vi "Teleop.vi"(10 "Match Info":T3={"Autonomous Elapsed Seconds"=0.0, "TeleOp Elapsed Seconds"=0.0, "Disabled Elapsed Seconds"=0.0, "Visited Autonomous"=FALSE, "Visited TeleOp"=FALSE, "Visited Disabled"=FALSE, "Autonomous Settings"={"Autonomous Style"=enum."Independent", "VI Refnum"=refnum}}, 11 "Call Context":T4) -> ()   [LabVIEW 2013]
doc: "This VI is called for each TeleOp packet received from the DS where the robot is not disabled. It is often used to read from the joysticks and update I/O or to update setpoints for timed control loops. It should complete and return within 20 milliseconds or it may miss DS packets."
uses:
  <vilib>/Rock Robotics/WPI/DriverStation/WPI_DriverStationDerivedRobotMode.ctl
  <vilib>/Rock Robotics/WPI/DriverStation/WPI_DriverStationMatch Info.ctl
  <vilib>/Rock Robotics/WPI/Solenoid/WPI_SolenoidValue.ctl
  Robot Global Data.vi
  <vilib>/Rock Robotics/WPI/Joystick/WPI_JoystickGetSetRefNum.vi
  <vilib>/Rock Robotics/WPI/Solenoid/WPI_SolenoidSetEnum.vi
  <vilib>/Rock Robotics/WPI/RobotDrive/WPI_RobotDriveGetSetRefNum.vi
  <vilib>/addons/control/pid/NI_PID_pid.lvlib
  <vilib>/addons/control/pid/pid.llb/PID (DBL).vi
panel:
  in  "Shooter Motor":dbl(slide) scale=-1.0..1.0
  in  "PID gains Anglerometer":T1={"proportional gain (Kc)"=1.0, "integral time (Ti, min)"=0.01, "derivative time (Td, min)"=0.0} {"derivative time (Td, min)" format="%.3f"; "integral time (Ti, min)" format="%.3f"; "proportional gain (Kc)" format="%.3f"}
  out "Shooter Angle":dbl
  out "Shooter At Target Angle":bool
  out "Cim Speed":dbl
  out "Time For Shooter":dbl
  in  "shooter state":T2(ring)
  out "Numeric 1":dbl(slide) scale=0.0..100.0
  out "Boolean 2":bool
  out "Boolean 1":bool
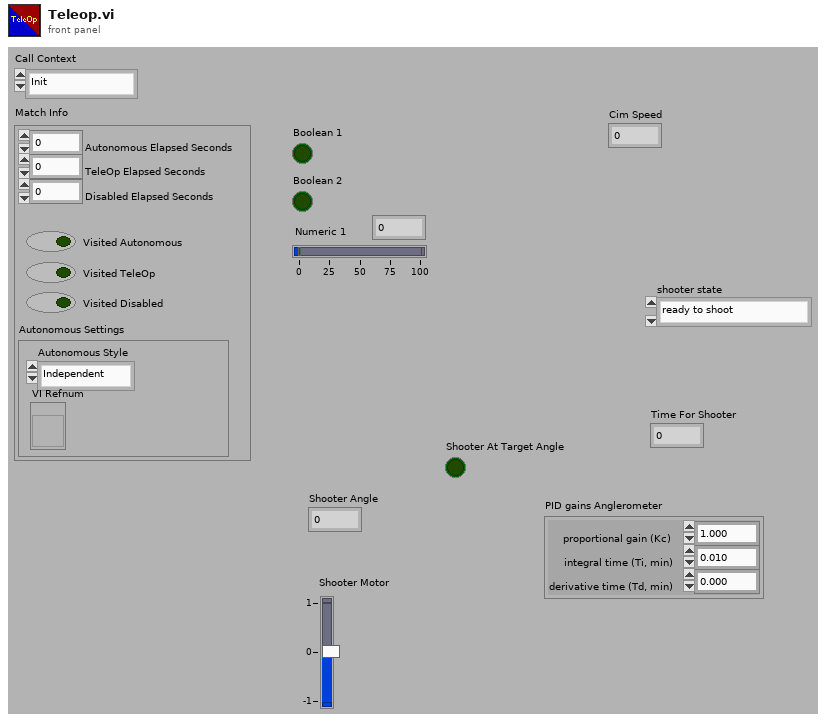
[diagram p1: front panel]
types:
  T1 = cluster{"proportional gain (Kc)":dbl, "integral time (Ti, min)":dbl, "derivative time (Td, min)":dbl}
  T2 = enum16{"ready to shoot", "shooting", "reloading"}
  T3 = typedef "WPI_DriverStationMatch Info.ctl" = cluster{"Autonomous Elapsed Seconds":dbl, "TeleOp Elapsed Seconds":dbl, "Disabled Elapsed Seconds":dbl, "Visited Autonomous":bool, "Visited TeleOp":bool, "Visited Disabled":bool, "Autonomous Settings":cluster{"Autonomous Style":enum16{"Iterative", "Independent"}, "VI Refnum":refnum<vi>}}
  T4 = typedef "WPI_DriverStationDerivedRobotMode.ctl" = enum16{"Init", "Execute", "Stop"}
  T5 = typedef "WPI_PWMDeviceRef.ctl" = cluster{"DeviceStatus":errorcluster, "Digital Module":T6, "PWM Channel":T7}
  T6 = typedef "FPGA_TypedefDigitalModule.ctl" = enum16{"Digital Module 1", "Digital Module 2"}
  T7 = typedef "FPGA_DIOPWMChannel.ctl" = enum8{"PWM 1", "PWM 2", "PWM 3", "PWM 4", "PWM 5", "PWM 6", "PWM 7", "PWM 8", "PWM 9", "PWM 10", "Invalid"}
  T8 = typedef "WPI_MotorControlDeviceRef.ctl" = cluster{"DeviceStatus":errorcluster, "Type":enum16{"PWM", "CAN"}, "PWM":cluster{"Digital Module":T6, "PWM Channel":T7, "DeadBand":T9}, "CAN":cluster{"Device Number":u8, "Control Mode":T10, "Semaphore":T11, "Max Vout":dbl}, "Invert":bool, "TransformRef":T12, "InvTransformRef":T12}
  T9 = typedef "WPI_PWMDeadband.ctl" = cluster{"Name":string, "maxPositivePwm":i32, "minPositivePwm":i32, "centerPwm":i32, "maxNegativePwm":i32, "minNegativePwm":i32, "angularRange":u16}
  T10 = typedef "WPI_CANJaguar_ControlMode.ctl" = enum8{"Percent VBus", "Current", "Speed", "Position", "Voltage"}
  T11 = typedef "Semaphore RefNum" = refnum<k1>
  T12 = typedef "WPI_PWMTransform_ConPane.ctl" = refnum<vi>
  T13 = typedef "WPI_RobotDriveDevRef.ctl" = cluster{"DevStatus":errorcluster, "Motors[]":T8[], "Square Inputs":bool, "Max Output":dbl, "Isochronous":bool}
  T14 = typedef "WPI_JoystickDevRef.ctl" = cluster{"Device":T15}
  T15 = typedef "WPI_JoystickDeviceEnum.ctl" = enum16{"USB 1", "USB 2", "USB 3", "USB 4", "Kinect 1", "Kinect 2"}
  T16 = typedef "WPI_JoystickButtonState.ctl" = cluster{"Button 1":bool, "Button 2":bool, "Button 3":bool, "Button 4":bool, "Button 5":bool, "Button 6":bool, "Button 7":bool, "Button 8":bool, "Button 9":bool, "Button 10":bool, "Button 11":bool, "Button 12":bool}
  T17 = cluster{"axis 1 (x)":dbl, "axis 2 (y)":dbl, "axis 3 (throttle)":dbl, "axis 4":dbl, "axis 5":dbl, "axis 6":dbl}
  T18 = typedef "WPI_SolenoidValue.ctl" = enum16{"Off", "On", "Forward", "Reverse"}
  T19 = typedef "WPI_SolenoidDevRef.ctl" = cluster{"DevStatus":errorcluster, "Solenoid Module":T20, "Forward Solenoid Channel":T21, "Reverse Solenoid Channel":T21}
  T20 = typedef "FPGA_TypedefSolenoidModule.ctl" = enum16{"Solenoid Module 1", "Solenoid Module 2"}
  T21 = typedef "WPI_SolenoidChannel.ctl" = enum8{"Solenoid 1", "Solenoid 2", "Solenoid 3", "Solenoid 4", "Solenoid 5", "Solenoid 6", "Solenoid 7", "Solenoid 8", "Invalid"}
  T22 = typedef "WPI_EncoderDevRef.ctl" = cluster{"DevStatus":errorcluster, "EncoderIndex":T23, "CounterIndex":T24, "DistancePerCount":dbl, "Decoding Type":T25}
  T23 = typedef "FPGA_EncoderIdx.ctl" = enum8{"Enc 0", "Enc 1", "Enc 2", "Enc 3", "Invalid"}
  T24 = typedef "FPGA_CounterCtrSystemIndex.ctl" = enum8{"Ctr 0", "Ctr 1", "Ctr 2", "Ctr 3", "Ctr 4", "Ctr 5", "Ctr 6", "Ctr 7", "Invalid"}
  T25 = typedef "WPI_EncoderType.ctl" = enum16{"1x", "2x", "4x"}
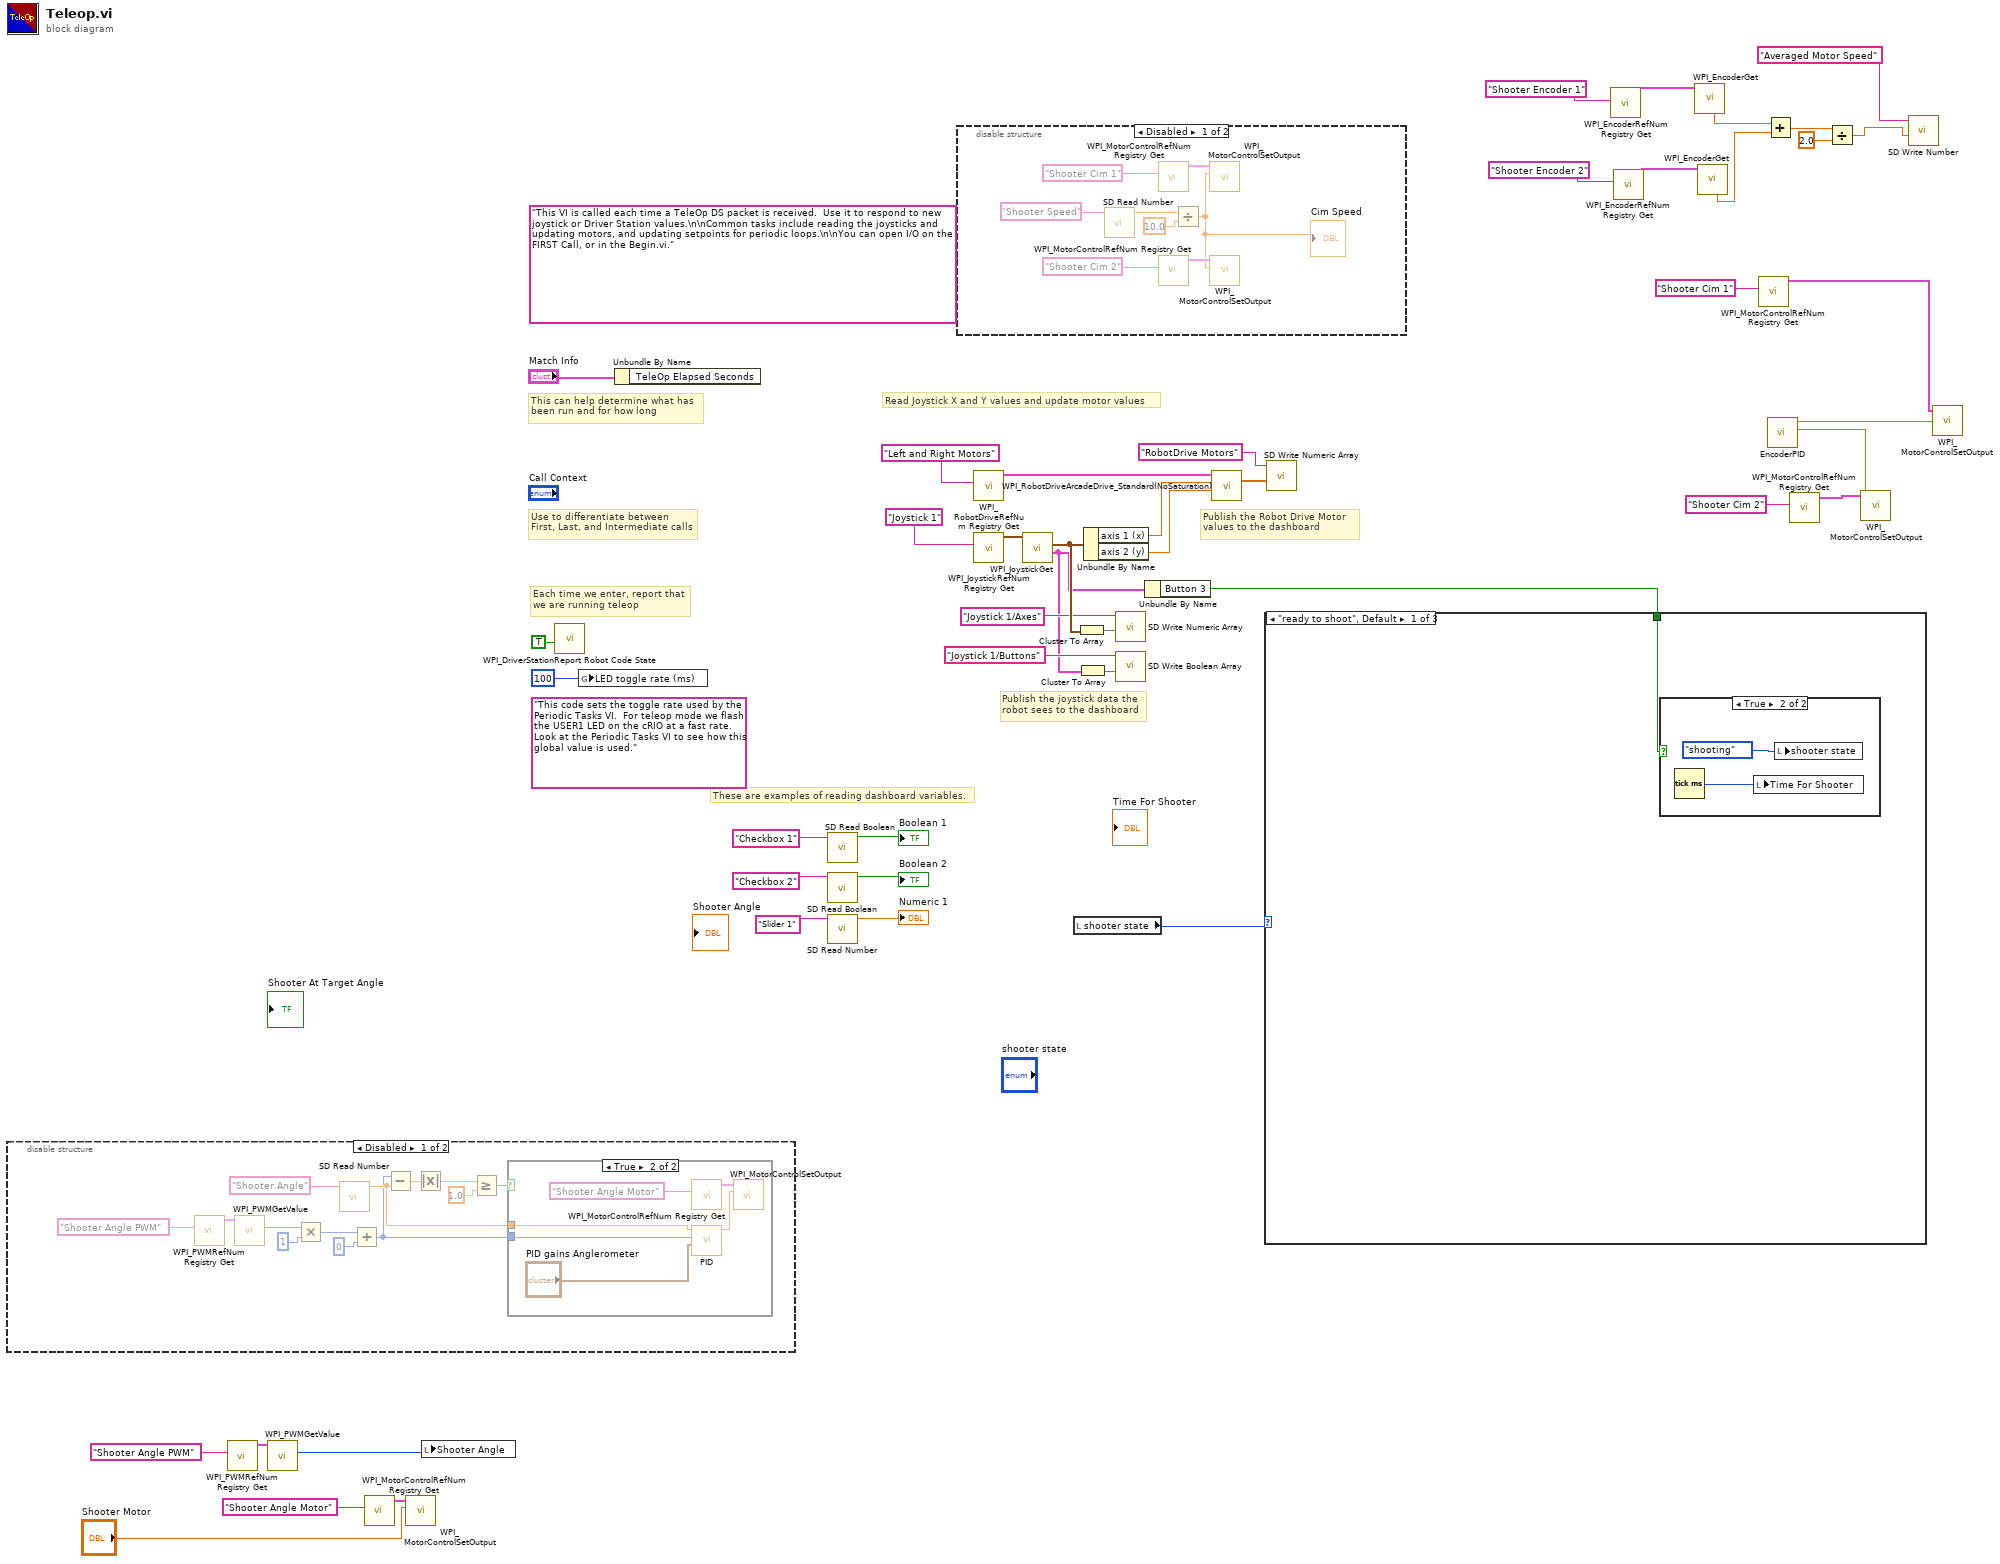
[diagram p0: block diagram]
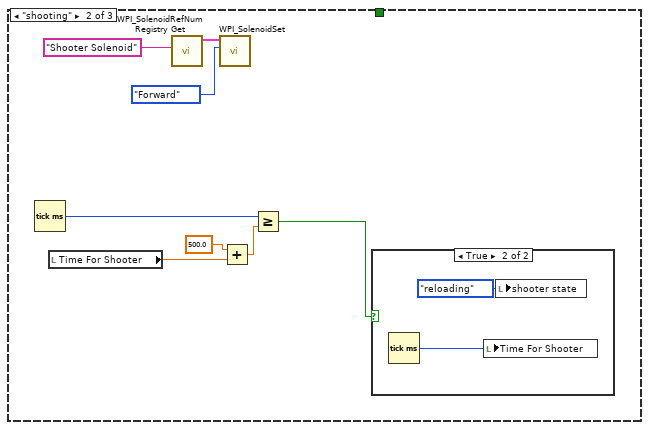
[diagram p6: hidden frame]
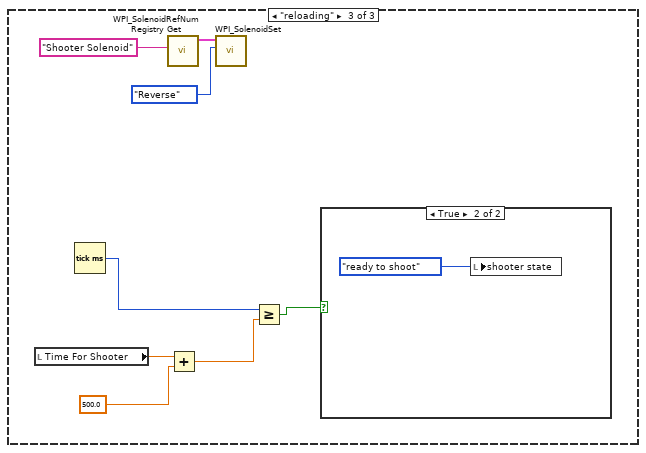
[diagram p8: hidden frame]
diagram:
  (unwired) "This code sets the toggle rate used by the Periodic Tasks VI.  For teleop mode we flash the USER1 LED on the cRIO at a fast rate.  Look at the Periodic Tasks VI to see how this global value is used."
  (unwired) "This VI is called each time a TeleOp DS packet is received.  Use it to respond to new joystick or Driver Station values.\n\nCommon tasks include reading the joysticks and updating motors, and updating setpoints for periodic loops.\n\nYou can open I/O on the FIRST Call, or in the Begin.vi."
  # "These are examples of reading dashboard variables."
  # "Publish the Robot Drive Motor\nvalues to the dashboard"
  # "Publish the joystick data the\nrobot sees to the dashboard"
  # "Each time we enter, report that\nwe are running teleop"
  # "Use to differentiate between\nFirst, Last, and Intermediate calls"
  # "This can help determine what has\nbeen run and for how long"
  # "Read Joystick X and Y values and update motor values"
  n1 = disable-structure shown="Disabled" {
    frame Disabled {
      n2 = call <vilib>:"WPI_PWMRefNum Registry Get.vi"("refnum name"="Shooter Angle PWM") -> ("PWMDeviceRef"=w60:T5)  [unwired: 9 in, 1 out]
      n3 = call <vilib>:"WPI_PWMGetValue.vi"("PWMDeviceRef"=w60) -> ("Value"=w57:u8)  [unwired: 8 in, 2 out]
      n4 = Multiply(x=w57, y=u8 1) -> (x*y=w55:u8)
      n5 = call <vilib>:"SD Read Number.vi"("Name"="Shooter Angle") -> ("Numeric"=w49:dbl)  [unwired: 8 in, 2 out]
      n6 = Add(x=w55, y=u8 0) -> (x+y=w48:u8)
      n7 = Subtract(x=w48, y=w49) -> (x-y=w53:dbl)
      n8 = Absolute Value(x=w53) -> (abs(x)=w52:dbl)
      n9 = Greater Or Equal?(x=w52, y=1.0) -> (x >= y?=w50:bool)
      n10 = case shown="True" w50 {
        tunnel: w49 -> [_ w66]
        tunnel: w48 -> [_ w65]
        frame False {
        }
        frame True {
          n11 = call <vilib>:"WPI_MotorControlRefNum Registry Get.vi"("refnum name"="Shooter Angle Motor") -> ("MotorControlDevRef"=w64:T8)  [unwired: 9 in, 1 out]
          n12 = call-poly <vilib>:"PID.vi"("PID gains"="PID gains Anglerometer", "process variable"=w65, "setpoint"=w66) -> ("output"=w62:dbl)  [unwired: 7 in, 1 out]
          n13 = call <vilib>:"WPI_MotorControlSetOutput.vi"("Output"=w62, "MotorControlDevRef"=w64) -> ()  [unwired: 7 in, 3 out]
        }
      }
    }
    frame Enabled {
    }
  }
  n14 = call <vilib>:"WPI_PWMRefNum Registry Get.vi"("refnum name"="Shooter Angle PWM") -> ("PWMDeviceRef"=w9:T5)  [unwired: 9 in, 1 out]
  n15 = call <vilib>:"WPI_PWMGetValue.vi"("PWMDeviceRef"=w9) -> ("Value"=w7:u8)  [unwired: 8 in, 2 out]
  n16 = call <vilib>:"WPI_MotorControlRefNum Registry Get.vi"("refnum name"="Shooter Angle Motor") -> ("MotorControlDevRef"=w6:T8)  [unwired: 9 in, 1 out]
  n17 = call <vilib>:"WPI_MotorControlSetOutput.vi"("Output"="Shooter Motor", "MotorControlDevRef"=w6) -> ()  [unwired: 7 in, 3 out]
  n18 = local write "Shooter Angle"(w7) -> ()
  n19 = call <vilib>:"WPI_DriverStationReport Robot Code State.vi"("TeleOp"=TRUE ("Autonomous")) -> ()  [unwired: 10 in, 1 out]
  n20 = global write "Robot Global Data.vi" "LED toggle rate (ms)"(u32 100 ("LED ms toggle rate")) -> ()
  n21 = Unbundle By Name("Match Info") -> ()  [unwired: 1 out]
  n22 = call <vilib>:"SD Read Boolean.vi"("Name"="Checkbox 1" ("refnum name")) -> ("Boolean"=→"Boolean 1":bool)  [unwired: 8 in, 2 out]
  n23 = call <vilib>:"SD Read Boolean.vi"("Name"="Checkbox 2" ("refnum name")) -> ("Boolean"=→"Boolean 2":bool)  [unwired: 8 in, 2 out]
  n24 = call <vilib>:"SD Read Number.vi"("Name"="Slider 1" ("refnum name")) -> ("Numeric"=→"Numeric 1":dbl)  [unwired: 8 in, 2 out]
  n25 = disable-structure shown="Disabled" {
    frame Disabled {
      n26 = call <vilib>:"SD Read Number.vi"("Name"="Shooter Speed") -> ("Numeric"=w69:dbl)  [unwired: 8 in, 2 out]
      n27 = call <vilib>:"WPI_MotorControlRefNum Registry Get.vi"("refnum name"="Shooter Cim 1") -> ("MotorControlDevRef"=w72:T8)  [unwired: 9 in, 1 out]
      n28 = call <vilib>:"WPI_MotorControlRefNum Registry Get.vi"("refnum name"="Shooter Cim 2") -> ("MotorControlDevRef"=w70:T8)  [unwired: 9 in, 1 out]
      n29 = Divide(x=w69, y=10.0) -> (x/y=w67:dbl)
      "Cim Speed" <- w67
      n30 = call <vilib>:"WPI_MotorControlSetOutput.vi"("Output"=w67, "MotorControlDevRef"=w72) -> ()  [unwired: 7 in, 3 out]
      n31 = call <vilib>:"WPI_MotorControlSetOutput.vi"("Output"=w67, "MotorControlDevRef"=w70) -> ()  [unwired: 7 in, 3 out]
    }
    frame Enabled {
    }
  }
  n32 = call <vilib>:"WPI_RobotDriveRefNum Registry Get.vi"("refnum name"="Left and Right Motors") -> ("RobotDriveDevRef"=w45:T13)  [unwired: 1 in, 9 out]
  n33 = call <vilib>:"WPI_JoystickRefNum Registry Get.vi"("refnum name"="Joystick 1") -> ("JoystickDevRef"=w41:T14)  [unwired: 1 in, 9 out]
  n34 = call <vilib>:"WPI_JoystickGet.vi"("JoystickDevRef"=w41) -> ("Buttons"=w2:T16, "Axes"=w36:T17)  [unwired: 1 in, 4 out]
  n35 = local read "shooter state"() -> (w25:T2)
  n36 = Cluster To Array(cluster=w36) -> (array=w35:dbl[])
  n37 = Cluster To Array(cluster=w2) -> (array=w38:bool[])
  n38 = Unbundle By Name(w36) -> ("axis 1 (x)"=w44:dbl, "axis 2 (y)"=w43:dbl)
  n39 = call <vilib>:"SD Write Numeric Array.vi"("Numeric Array"=w35, "Name"="Joystick 1/Axes") -> ()  [unwired: 8 in, 2 out]
  n40 = call <vilib>:"SD Write Boolean Array.vi"("Boolean Array"=w38, "Name"="Joystick 1/Buttons") -> ()  [unwired: 8 in, 2 out]
  n41 = Unbundle By Name(w2) -> ("Button 3"=w1:bool)
  n42 = call <vilib>:"WPI_RobotDriveArcadeDrive_Standard(NoSaturation).vi"("Y axis value"=w43, "X axis value"=w44, "RobotDriveDevRef"=w45) -> ("Motor Values"=w32:dbl[])  [unwired: 1 in, 7 out]
  n43 = case shown="\"ready to shoot\", Default" w25 {
    tunnel: w1 -> [w75 _ _]
    frame "ready to shoot", Default {
      n44 = case shown="True" w75 {
        frame False {
        }
        frame True {
          n45 = Tick Count (ms)() -> (millisecond timer value=w76:u32)
          n46 = local write "Time For Shooter"(w76) -> ()
          n47 = local write "shooter state"(T2."shooting" ("shooter state")) -> ()
        }
      }
    }
    frame "shooting" {
      n48 = Tick Count (ms)() -> (millisecond timer value=w78:u32)
      n49 = local read "Time For Shooter"() -> (w80:dbl)
      n50 = call <vilib>:"WPI_SolenoidRefNum Registry Get.vi"("refnum name"="Shooter Solenoid") -> ("SolenoidDevRef"=w84:T19)  [unwired: 9 in, 1 out]
      n51 = call-poly <vilib>:"WPI_SolenoidSet.vi"("Value"=WPI_SolenoidValue."Forward", "SolenoidDevRef"=w84) -> ()  [unwired: 8 in, 2 out]
      n52 = Add(x=500.0, y=w80) -> (x+y=w79:dbl)
      n53 = Greater Or Equal?(x=w78, y=w79) -> (x >= y?=w82:bool)
      n54 = case shown="True" w82 {
        frame False {
        }
        frame True {
          n55 = Tick Count (ms)() -> (millisecond timer value=w86:u32)
          n56 = local write "Time For Shooter"(w86) -> ()
          n57 = local write "shooter state"(T2."reloading" ("shooter state")) -> ()
        }
      }
    }
    frame "reloading" {
      n58 = local read "Time For Shooter"() -> (w90:dbl)
      n59 = Tick Count (ms)() -> (millisecond timer value=w92:u32)
      n60 = call <vilib>:"WPI_SolenoidRefNum Registry Get.vi"("refnum name"="Shooter Solenoid") -> ("SolenoidDevRef"=w94:T19)  [unwired: 9 in, 1 out]
      n61 = Add(x=w90, y=500.0) -> (x+y=w88:dbl)
      n62 = call-poly <vilib>:"WPI_SolenoidSet.vi"("Value"=WPI_SolenoidValue."Reverse", "SolenoidDevRef"=w94) -> ()  [unwired: 8 in, 2 out]
      n63 = Greater Or Equal?(x=w92, y=w88) -> (x >= y?=w91:bool)
      n64 = case shown="True" w91 {
        frame False {
        }
        frame True {
          n65 = local write "shooter state"(T2."ready to shoot" ("shooter state")) -> ()
        }
      }
    }
  }
  n66 = call <vilib>:"SD Write Numeric Array.vi"("Numeric Array"=w32, "Name"="RobotDrive Motors") -> ()  [unwired: 8 in, 2 out]
  n67 = call <vilib>:"WPI_EncoderRefNum Registry Get.vi"("refnum name"="Shooter Encoder 1") -> ("EncoderDevRef"=w23:T22)  [unwired: 9 in, 1 out]
  n68 = call <vilib>:"WPI_EncoderRefNum Registry Get.vi"("refnum name"="Shooter Encoder 2") -> ("EncoderDevRef"=w21:T22)  [unwired: 9 in, 1 out]
  n69 = call <vilib>:"WPI_EncoderGet.vi"("EncoderDevRef"=w23) -> ("Rate"=w15:dbl)  [unwired: 5 in, 5 out]
  n70 = call <vilib>:"WPI_EncoderGet.vi"("EncoderDevRef"=w21) -> ("Rate"=w16:dbl)  [unwired: 5 in, 5 out]
  n71 = call <vilib>:"WPI_MotorControlRefNum Registry Get.vi"("refnum name"="Shooter Cim 1") -> ("MotorControlDevRef"=w13:T8)  [unwired: 9 in, 1 out]
  n72 = Add(x=w15, y=w16) -> (x+y=w20:dbl)
  n73 = call "EncoderPID.vi"() -> ("PID 2 Output"=w3:dbl, "PID 1 Output"=w10:dbl)  [unwired: 10 in]
  n74 = call <vilib>:"WPI_MotorControlRefNum Registry Get.vi"("refnum name"="Shooter Cim 2") -> ("MotorControlDevRef"=w11:T8)  [unwired: 9 in, 1 out]
  n75 = Divide(x=w20, y=2.0) -> (x/y=w18:dbl)
  n76 = call <vilib>:"WPI_MotorControlSetOutput.vi"("Output"=w3, "MotorControlDevRef"=w11) -> ()  [unwired: 7 in, 3 out]
  n77 = call <vilib>:"SD Write Number.vi"("Numeric"=w18, "Name"="Averaged Motor Speed") -> ()  [unwired: 8 in, 2 out]
  n78 = call <vilib>:"WPI_MotorControlSetOutput.vi"("Output"=w10, "MotorControlDevRef"=w13) -> ()  [unwired: 7 in, 3 out]
